vi "Data Store.vi"(8 "error in (no error)":errorcluster, 10 "new weather data":T1, 11 "action":u16(ring) items=["Initialize Data Store", "Destroy Data Store", "Clear Data", "Append Data", "Get Last Data", "Get All Data"]) -> (0 "error out":errorcluster, 2 "weather data out":T1[](array[typedef]))   [LabVIEW 2023, in "Weather Data.lvlib"]
doc: "Stores and provides access to weather data. This VI uses a functional global variable to provide access for both the weather simulator application and the web service included with the application. Because it is non-reentrant and reserved by the main application VI, the data is available throughout the application."
uses:
  Weather Data.lvlib
  Weather Data.ctl
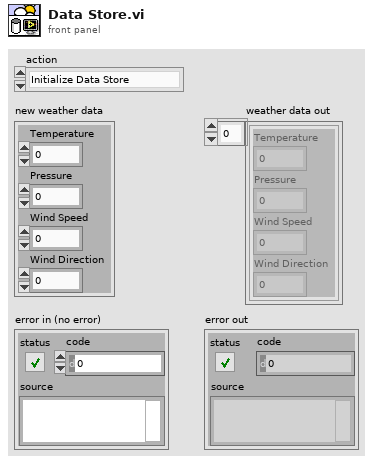
[diagram p1: front panel]
types:
  T1 = typedef "Weather Data.lvlib/Weather Data.ctl" = cluster{"Temperature":dbl, "Pressure":dbl, "Wind Speed":dbl, "Wind Direction":dbl}
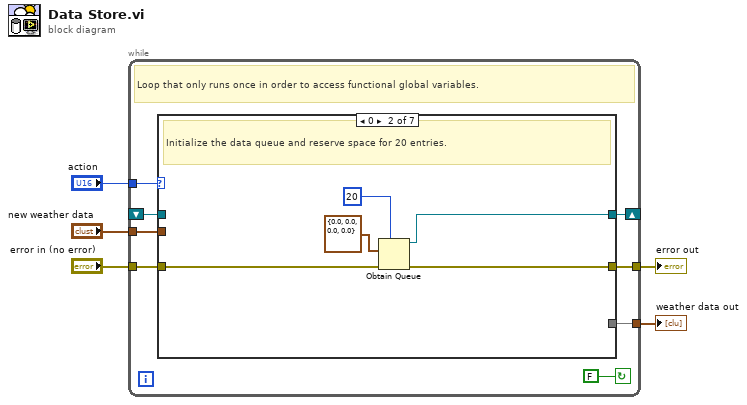
[diagram p0: block diagram]
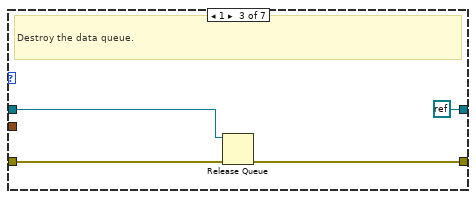
[diagram p3: hidden frame]
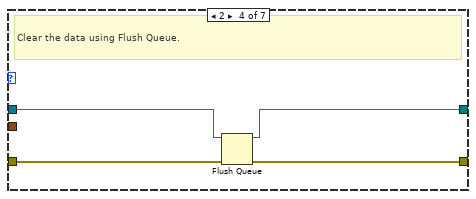
[diagram p4: hidden frame]
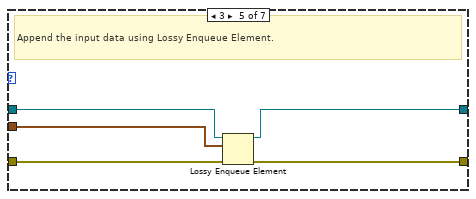
[diagram p5: hidden frame]
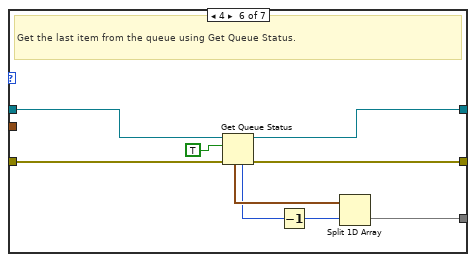
[diagram p6: hidden frame]
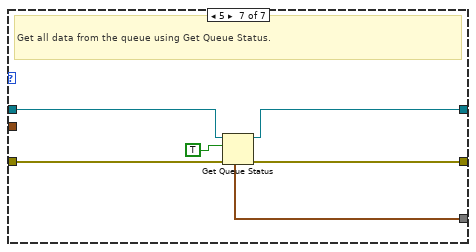
[diagram p7: hidden frame]
diagram:
  n1 = while {
    tunnel: "action" -> [w13]
    shift-right: [w11] -> _
    shift-left: _ -> [w10]
    tunnel: "error in (no error)" -> [w9]
    tunnel: [w8] -> w3
    tunnel: "new weather data" -> [w7]
    tunnel: [w6] -> w1
    stop <- FALSE continue-if-true
    # "Loop that only runs once in order to access functional global variables."
    n2 = case shown="0" w13 {
      tunnel: [w15 w20 refnum<k0> refnum w27 w30 w39 w45] -> w11
      tunnel: w10 -> [w15 _ w22 w28 w31 w40 w46]
      tunnel: w9 -> [w14 w17 w24 w26 w33 w42 w48]
      tunnel: [w14 w16 w23 w25 w32 w41 w47] -> w8
      tunnel: w7 -> [_ _ _ _ w29 _ _]
      tunnel: [_ _ _ _ _ w34 w43] -> w6
      frame Default {
        # "Invalid action."
      }
      frame 0 {
        # "Initialize the data queue and reserve space for 20 entries."
        n3 = Obtain Queue(max queue size (-1, unlimited)=20, element data type=T1 {"Temperature"=0.0, "Pressure"=0.0, "Wind Speed"=0.0, "Wind Direction"=0.0} ("Weather Data"), error in (no error)=w17) -> (queue out=w20:refnum<queue>, error out=w16:errorcluster)  [unwired: 2 in, 1 out]
      }
      frame 1 {
        # "Destroy the data queue."
        n4 = Release Queue(queue=w22, error in (no error)=w24) -> (error out=w23:errorcluster)  [unwired: 1 in, 2 out]
      }
      frame 2 {
        # "Clear the data using Flush Queue."
        n5 = Flush Queue(queue=w28, error in (no error)=w26) -> (queue out=w27:refnum<queue>, error out=w25:errorcluster)  [unwired: 1 out]
      }
      frame 3 {
        # "Append the input data using Lossy Enqueue Element."
        n6 = Lossy Enqueue Element(queue=w31, element=w29, error in (no error)=w33) -> (queue out=w30:refnum<queue>, error out=w32:errorcluster)  [unwired: 2 out]
      }
      frame 4 {
        # "Get the last item from the queue using Get Queue Status."
        n7 = Get Queue Status(queue=w40, return elements? (F)=TRUE, error in (no error)=w42) -> (queue out=w39:refnum<queue>, error out=w41:errorcluster, # elements in queue=w36:i32, elements=w37:T1[])  [unwired: 4 out]
        n8 = Decrement(x=w36) -> (x-1=w35:i32)
        n9 = Split 1D Array(array=w37, index=w35) -> (second subarray=w34:T1[])  [unwired: 1 out]
      }
      frame 5 {
        # "Get all data from the queue using Get Queue Status."
        n10 = Get Queue Status(queue=w46, return elements? (F)=TRUE, error in (no error)=w48) -> (queue out=w45:refnum<queue>, error out=w47:errorcluster, elements=w43:T1[])  [unwired: 5 out]
      }
    }
  }
  "error out" <- w3
  "weather data out" <- w1
